vi "Dispense.vi"(8 "error in (no error)":errorcluster, 10 "Bottom Pin":tag="A/PWM1", 11 "Top Pin":tag="A/PWM0") -> (0 "error out":errorcluster, 3 "Finished":bool)   [LabVIEW 2014]
uses:
  Controls/Dispenser Functions.ctl
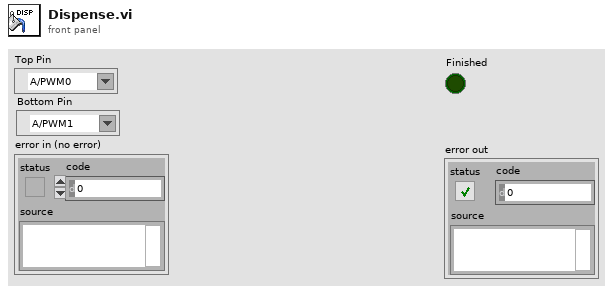
[diagram p1: front panel]
types:
  T1 = typedef "Dispenser Functions.ctl" = enum16{"Open Top", "Close Top", "Close Bottom", "Open Bottom"}
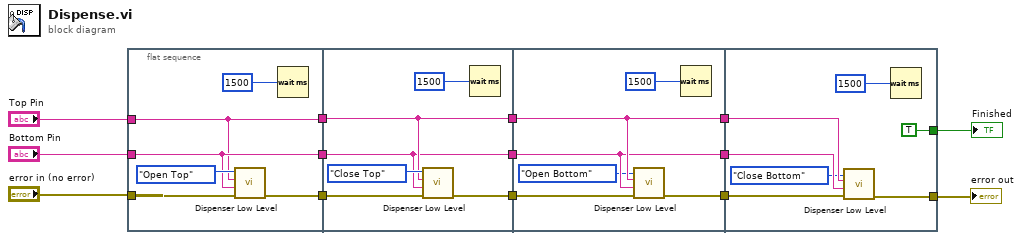
[diagram p0: block diagram]
diagram:
  n1 = flat-sequence {
    tunnel: "Bottom Pin" -> [w16]
    tunnel: [w16] -> w13
    tunnel: "Top Pin" -> [w15]
    tunnel: [w15] -> w9
    tunnel: "error in (no error)" -> [w19]
    tunnel: [w18] -> w6
    tunnel: w13 -> [w22]
    tunnel: [w22] -> w12
    tunnel: w9 -> [w23]
    tunnel: [w23] -> w8
    tunnel: w6 -> [w24]
    tunnel: [w21] -> w4
    tunnel: w12 -> [w30]
    tunnel: [w30] -> w11
    tunnel: w8 -> [w31]
    tunnel: [w31] -> w7
    tunnel: w4 -> [w28]
    tunnel: [w27] -> w3
    tunnel: w11 -> [w35]
    tunnel: w7 -> [w36]
    tunnel: w3 -> [w38]
    tunnel: [w37] -> w2
    tunnel: [TRUE ("Finished")] -> w1
    frame #0 {
      n2 = call "Dispenser Low Level.vi"("error in (no error)"=w19, "Bottom Pin"=w16, "Top Pin"=w15, "Function"=Dispenser_Functions."Open Top") -> ("error out"=w18:errorcluster)  [unwired: 7 in]
      n3 = Wait (ms)(milliseconds to wait=u32 1500) -> ()  [unwired: 1 out]
    }
    frame #1 {
      n4 = call "Dispenser Low Level.vi"("error in (no error)"=w24, "Bottom Pin"=w22, "Top Pin"=w23, "Function"=Dispenser_Functions."Close Top") -> ("error out"=w21:errorcluster)  [unwired: 7 in]
      n5 = Wait (ms)(milliseconds to wait=u32 1500) -> ()  [unwired: 1 out]
    }
    frame #2 {
      n6 = call "Dispenser Low Level.vi"("error in (no error)"=w28, "Bottom Pin"=w30, "Top Pin"=w31, "Function"=Dispenser_Functions."Open Bottom") -> ("error out"=w27:errorcluster)  [unwired: 7 in]
      n7 = Wait (ms)(milliseconds to wait=u32 1500) -> ()  [unwired: 1 out]
    }
    frame #3 {
      n8 = call "Dispenser Low Level.vi"("error in (no error)"=w38, "Bottom Pin"=w35, "Top Pin"=w36, "Function"=Dispenser_Functions."Close Bottom") -> ("error out"=w37:errorcluster)  [unwired: 7 in]
      n9 = Wait (ms)(milliseconds to wait=u32 1500) -> ()  [unwired: 1 out]
    }
  }
  "error out" <- w2
  "Finished" <- w1
